vi "Add AOIs overlay to image.vi"(6 "Font, Size & Style":T1={"Desired Font (Application)"=enum."Application Font", "[User-specified Font]"={"Font Name"="", "Size"=12, "Strikeout?"=FALSE, "Italic?"=FALSE, "Underline?"=FALSE, "Outline?"=FALSE, "Shadow?"=FALSE, "Bold?"=FALSE, "Rotation Angle"=0.0}, "Horizontal Alignment"=0, "Vertical Alignment"=0} {"Vertical Alignment" items=["Bottom", "Top", "Baseline"]; "Horizontal Alignment" items=["Left", "Center", "Right"]; "[User-specified Font]"."Rotation Angle" format="%.2f"}, 7 "Color":u32(colorbox)=16711680, 8 "error in (no error)":errorcluster, 9 "Current frame number\n(starting with 1)":u32, 10 "Overlay on?":bool=TRUE, 11 "Image Src":T2) -> (0 "error out":errorcluster, 3 "Image Dst":T2)   [LabVIEW 2016]
doc: "Draws AOIs listed in the global multiple AOI list into the overlay."
uses:
  <vilib>/vision/Image Controls.llb/IMAQ Image.ctl
  AOI List Globals.vi
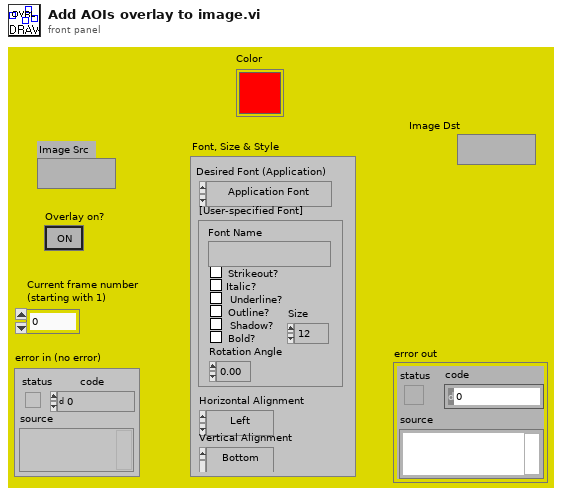
[diagram p1: front panel]
types:
  T1 = cluster{"Desired Font (Application)":enum16{"User-specified Font", "Application Font", "System Font", "Dialog Font"}, "[User-specified Font]":cluster{"Font Name":string, "Size":i16, "Strikeout?":bool, "Italic?":bool, "Underline?":bool, "Outline?":bool, "Shadow?":bool, "Bold?":bool, "Rotation Angle":dbl}, "Horizontal Alignment":i16, "Vertical Alignment":i16}
  T2 = typedef "IMAQ Image.ctl" = refnum<image>
  T3 = cluster{"Left":i32, "Top":i32, "Right":i32, "Bottom":i32}
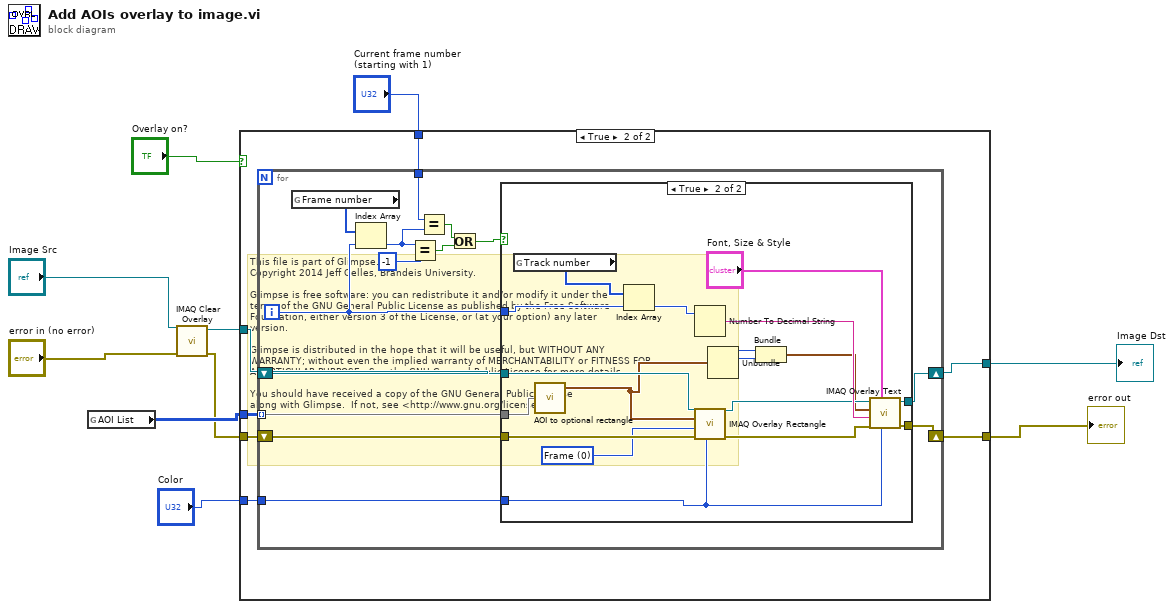
[diagram p0: block diagram]
diagram:
  # "This file is part of Glimpse. \nCopyright 2014 Jeff Gelles, Brandeis University.    \n\nGlimpse is free software: you can redistribute it and/or modify it under the \nterms of the GNU General Public License as published by the Free Software \nFoundation, either version 3 of the License, or (at your option) any later \nversion.\n\nGlimpse is distributed in the hope that it will be useful, but WITHOUT ANY \nWARRANTY; without even the implied warranty of MERCHANTABILITY or FITNESS FOR \nA PARTICULAR PURPOSE.  See the GNU General Public License for more details.\n\nYou should have received a copy of the GNU General Public License\nalong with Glimpse.  If not, see <http://www.gnu.org/licenses/>."
  n1 = global read "AOI List Globals.vi" "AOI List"() -> (w10:u16[][])
  n2 = call "IMAQ Clear Overlay"("error in (no error)"="error in (no error)", "Image"="Image Src") -> ("error out"=w7:errorcluster, "Image Out"=w8:T2)  [unwired: 2 in, 6 out]
  n3 = case shown="True" "Overlay on?" {
    tunnel: w10 -> [_ w19]
    tunnel: w8 -> [w12 w18]
    tunnel: w7 -> [w11 w17]
    tunnel: "Color" -> [_ w16]
    tunnel: [w12 w15] -> w4
    tunnel: [w11 w14] -> w3
    tunnel: "Current frame number\n(starting with 1)" -> [_ w13]
    frame False {
    }
    frame True {
      n4 = for {
        tunnel: w19 -> [w29] mode=indexing
        shift-right: [w30] -> w14
        shift-left: w17 -> [w31]
        shift-right: [w32] -> w15
        shift-left: w18 -> [w33]
        tunnel: w16 -> [w28]
        tunnel: w13 -> [w21]
        i -> [w26]
        n5 = global read "AOI List Globals.vi" "Frame number"() -> (w27:i32[])
        n6 = Index Array(array=w27, index=w26) -> (element=w22:i32)
        n7 = Equal?(x=w22, y=-1) -> (x = y?=w24:bool)
        n8 = Equal?(x=w21, y=w22) -> (x = y?=w23:bool)
        n9 = Or(x=w23, y=w24) -> (x .or. y?=w20:bool)
        n10 = case shown="True" w20 {
          tunnel: w33 -> [w35 w53]
          tunnel: [w35 w52] -> w32
          tunnel: w31 -> [w34 w50]
          tunnel: [w34 w48] -> w30
          tunnel: w29 -> [_ w46]
          tunnel: w28 -> [_ w39]
          tunnel: w26 -> [_ w36]
          frame False {
          }
          frame True {
            w45 = u32 0 items=["Frame", "Fill", "Highlight"] ("Drawing Mode (Frame)")
            n11 = global read "AOI List Globals.vi" "Track number"() -> (w37:u16[])
            n12 = call "AOI to optional rectangle.vi"("x1, y1, x2, y2 with origin (0, 0)"=w46) -> ("Rectangle Out"=w43:T3)  [unwired: 4 out]
            n13 = Index Array(array=w37, index=w36) -> (element=w38:u16)
            n14 = Number To Decimal String(number=w38) -> (decimal integer string=w51:string)  [unwired: 1 out]
            n15 = call "IMAQ Overlay Rectangle"("Color"=w39, "error in (no error)"=w50, "Drawing Mode (Frame)"=w45, "Rectangle"=w43, "Image"=w53) -> ("error out"=w49:errorcluster, "Image Out"=w47:T2)  [unwired: 1 in, 4 out]
            n16 = Unbundle(w43) -> ("Left"=w41:i32, "Top"=w42:i32)  [unwired: 2 out]
            n17 = Bundle("Left"=w41, "Top"=w42) -> (w40:cluster{"Left":i32, "Top":i32})  [unwired: 1 out]
            n18 = call "IMAQ Overlay Text"("Text Color (black)"=w39, "Font, Size & Style"="Font, Size & Style", "error in (no error)"=w49, "String"=w51, "Origin"=w40, "Image"=w47) -> ("error out"=w48:errorcluster, "Image Out"=w52:T2)  [unwired: 2 in, 2 out]
          }
        }
      }
    }
  }
  "Image Dst" <- w4
  "error out" <- w3
